vi "get_packed_len.vi"(3 "error in":errorcluster, 5 "p":u64) -> (0 "error out":errorcluster, 1 "len":u32, 2 "p out":u64)   [LabVIEW 2019, in "msgpack.lvlib"]
doc: "Returns a pointer to the current msgpack buffer and the length of the current packed string; intended for passing on directly to other C API.\n\nUse copy_packed_data if you wish to access the data from labview"
uses:
  msgpack.lvlib
  msgpackalt.dll
panel:
  # "msgpack"
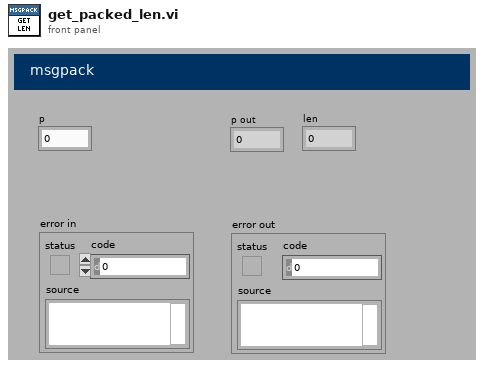
[diagram p1: front panel]
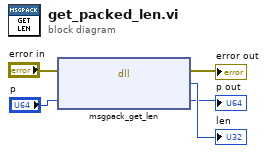
[diagram p0: block diagram]
diagram:
  n1 = dll-call lib="C:/Users/Patrick/Documents/GitHub/Instrument-Framework/lvsrc/SMOs/JSON-RPC-2019/lv-venv/lv.lib/vi.lib/addons/msgpack/msgpackalt.dll" fn="msgpack_get_len"(error in="error in", "p"="p") -> (error out=→"error out":errorcluster, "return type"=→"len":u32, "p"=→"p out":u64)  [unwired: 2 in, 1 out]
